vi "Save Parametric Data to csv.vi"(0 "Filepath":path=path "C:/Users/Eddie.Rickey/Desktop/Test Data", 2 "Test Information":T4={"Exp Name"="Cold Switching", "Lot"="0233A", "Wafer"="15", "Die Type"="L22", "Die X "="6", "Die Y"="8", "Exp"="1", "Die X_Y"="8"}, 3 "Parametric Calculated Values":T5={"Voltage Calculated Values"={"P1_VPD_C"=0.0, "P2_VPD_C"=0.0, "P1_VPD_Rel_C"=0.0, "P2_VPD_Rel_C"=0.0}, "Resistance Calculated Values"={"Rc_free"=0.0, "Rc_first"=0.0, "Rc_vmax"=0.0, "Rc_last"=0.0, "Rc_end"=0.0, "VPD_R"=0.0, "VPD_Rel_R"=0.0}, "Capacitance Calculated Values"={"P1_CPD_free"=0.0, "P2_CPD_free"=0.0, "P1_CPD_vmax"=0.0, "P2_CPD_vmax"=0.0, "P1_CPD_first"=0.0, "P2_CPD_first"=0.0, "P1_CPD_last"=0.0, "P2_CPD_last"=0.0, "P1_CPD_end"=0.0, "P2_CPD_end"=0.0, "P1_CPD_max"=0.0, "P2_CPD_max "=0.0, "CPD_Free"=0.0, "CPD_First"=0.0, "CPD_max"=0.0, "CPD_Last"=0.0, "CPD_End"=0.0, "CPD_vmax"=0.0}, "Cap Calc Arrays"={"CPD_sum"=[], "P2_CPD@V"=[], "P1_CPD@V"=[], "Specific Voltages"=[32.0, 36.0]}, "Resistance Array Calc"={"RC@V"=[]}, "TN4 Calc"={"P1_TN4_ACT"=0.0, "P2_TN4_ACT "=0.0, "VPD_R_2"=0.0, "DVR"=0.0}, "Corrected_Capacitance Calculated Values"={"P1_CPD_free"=0.0, "P2_CPD_free"=0.0, "P1_CPD_vmax"=0.0, "P2_CPD_vmax"=0.0, "P1_CPD_first"=0.0, "P2_CPD_first"=0.0, "P1_CPD_last"=0.0, "P2_CPD_last"=0.0, "P1_CPD_end"=0.0, "P2_CPD_end"=0.0, "P1_CPD_max"=0.0, "P2_CPD_max "=0.0, "CPD_Free"=0.0, "CPD_First"=0.0, "CPD_max"=0.0, "CPD_Last"=0.0, "CPD_End"=0.0, "CPD_vmax"=0.0}}, 4 "Date Cluster":T3, 5 "Error In":errorcluster, 6 "Cal Measurements":T1 {"Port 3 Capacitance" format="%#_6p"; "Port 2 Capacitance" format="%#_6p"; "Port 1 Capacitance" format="%#_6p"}, 8 "Additional Data":T2, 10 "Meas Type":string) -> (19 "Error Out":errorcluster)   [LabVIEW 2013]
uses:
  Controls/Parametric Calculated Values.ctl
  Controls/Voltage Calculated Values.ctl
  Controls/Resistance Individual Calculated Values.ctl
  Controls/Capacitance Individual Calculated Values.ctl
  Controls/Capacitance Array Calculated Values.ctl
  Controls/Resistance Array Calculated Values.ctl
  Controls/TN4 Calc.ctl
  Controls/Corrected_Capacitance Individual Calculated Values.ctl
  Controls/Test Information.ctl
  Controls/Date Control.ctl
  Controls/Additional Data.ctl
  Controls/ENA_Marker Measurements.ctl
  <vilib>/Utility/file.llb/Write To Spreadsheet File (string).vi
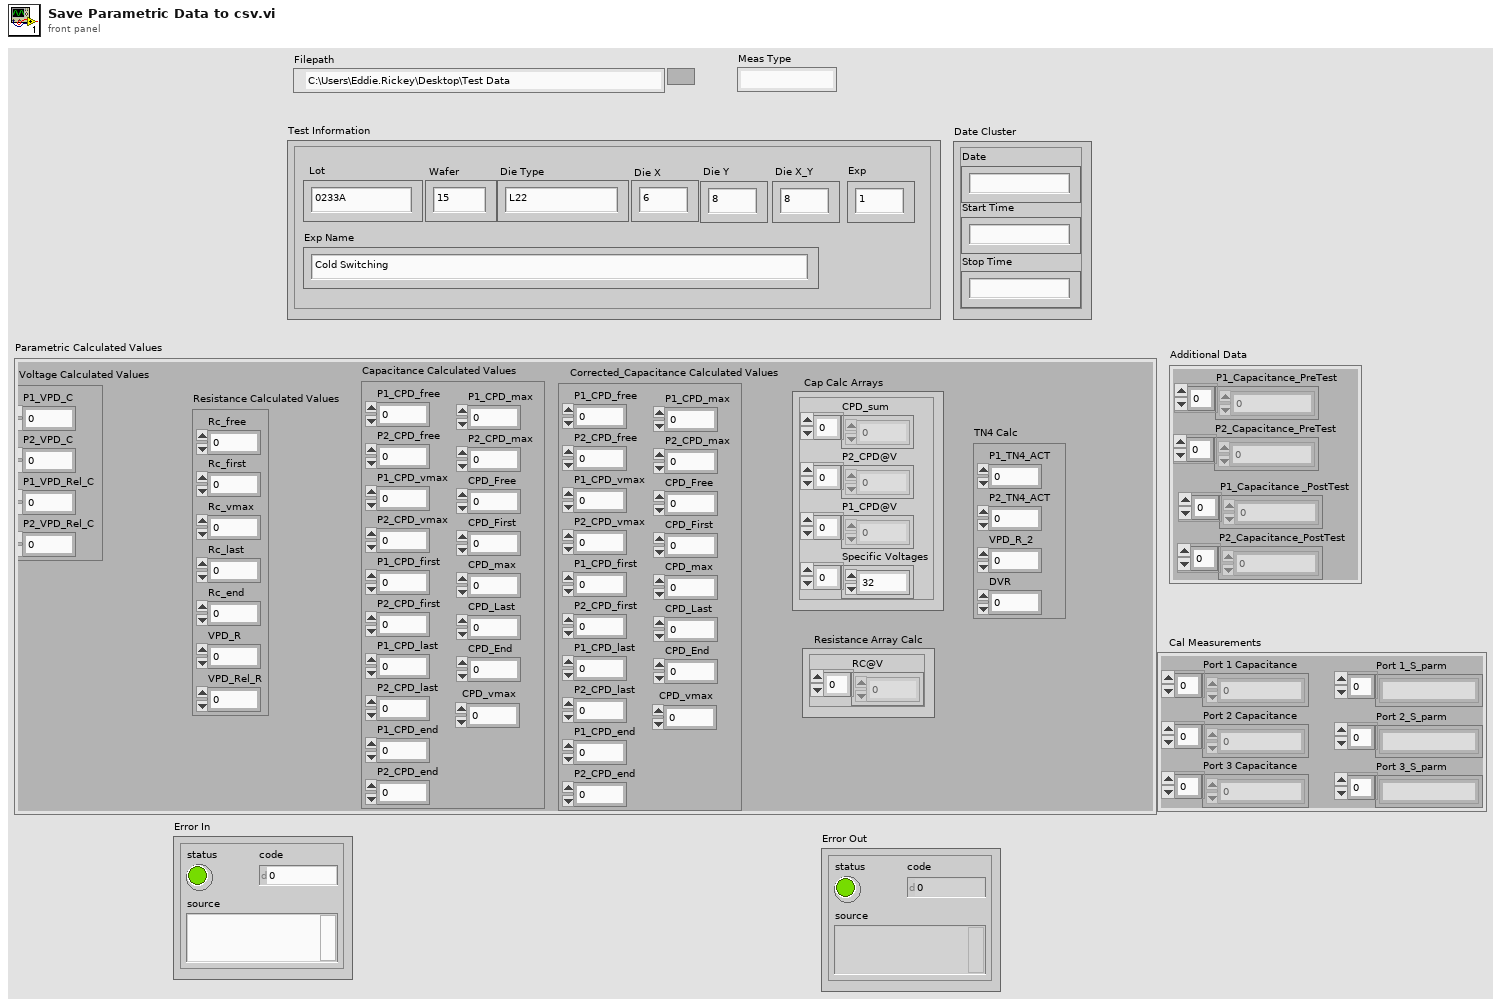
[diagram p1: front panel]
types:
  T1 = typedef "ENA_Marker Measurements.ctl" = cluster{"Port 1 Capacitance":dbl[], "Port 2 Capacitance":dbl[], "Port 3 Capacitance":dbl[], "Port 1_S_parm":string[], "Port 2_S_parm":string[], "Port 3_S_parm":string[]}
  T2 = typedef "Additional Data.ctl" = cluster{"P2_Capacitance_PostTest":dbl[], "P1_Capacitance _PostTest":dbl[], "P1_Capacitance_PreTest":dbl[], "P2_Capacitance_PreTest":dbl[]}
  T3 = typedef "Date Control.ctl" = cluster{"Date":string, "Start Time":string, "Stop Time":string}
  T4 = typedef "Test Information.ctl" = cluster{"Exp Name":string, "Lot":string, "Wafer":string, "Die Type":string, "Die X ":string, "Die Y":string, "Exp":string, "Die X_Y":string}
  T5 = typedef "Parametric Calculated Values.ctl" = cluster{"Voltage Calculated Values":T6, "Resistance Calculated Values":T7, "Capacitance Calculated Values":T8, "Cap Calc Arrays":T9, "Resistance Array Calc":T10, "TN4 Calc":T11, "Corrected_Capacitance Calculated Values":T12}
  T6 = typedef "Voltage Calculated Values.ctl" = cluster{"P1_VPD_C":dbl, "P2_VPD_C":dbl, "P1_VPD_Rel_C":dbl, "P2_VPD_Rel_C":dbl}
  T7 = typedef "Resistance Individual Calculated Values.ctl" = cluster{"Rc_free":dbl, "Rc_first":dbl, "Rc_vmax":dbl, "Rc_last":dbl, "Rc_end":dbl, "VPD_R":dbl, "VPD_Rel_R":dbl}
  T8 = typedef "Capacitance Individual Calculated Values.ctl" = cluster{"P1_CPD_free":dbl, "P2_CPD_free":dbl, "P1_CPD_vmax":dbl, "P2_CPD_vmax":dbl, "P1_CPD_first":dbl, "P2_CPD_first":dbl, "P1_CPD_last":dbl, "P2_CPD_last":dbl, "P1_CPD_end":dbl, "P2_CPD_end":dbl, "P1_CPD_max":dbl, "P2_CPD_max ":dbl, "CPD_Free":dbl, "CPD_First":dbl, "CPD_max":dbl, "CPD_Last":dbl, "CPD_End":dbl, "CPD_vmax":dbl}
  T9 = typedef "Capacitance Array Calculated Values.ctl" = cluster{"CPD_sum":dbl[], "P2_CPD@V":dbl[], "P1_CPD@V":dbl[], "Specific Voltages":dbl[]}
  T10 = typedef "Resistance Array Calculated Values.ctl" = cluster{"RC@V":dbl[]}
  T11 = typedef "TN4 Calc.ctl" = cluster{"P1_TN4_ACT":dbl, "P2_TN4_ACT ":dbl, "VPD_R_2":dbl, "DVR":dbl}
  T12 = typedef "Corrected_Capacitance Individual Calculated Values.ctl" = cluster{"P1_CPD_free":dbl, "P2_CPD_free":dbl, "P1_CPD_vmax":dbl, "P2_CPD_vmax":dbl, "P1_CPD_first":dbl, "P2_CPD_first":dbl, "P1_CPD_last":dbl, "P2_CPD_last":dbl, "P1_CPD_end":dbl, "P2_CPD_end":dbl, "P1_CPD_max":dbl, "P2_CPD_max ":dbl, "CPD_Free":dbl, "CPD_First":dbl, "CPD_max":dbl, "CPD_Last":dbl, "CPD_End":dbl, "CPD_vmax":dbl}
  T13 = enum16{"open", "replace", "create", "open or create", "replace or create", "replace or create with confirmation"}
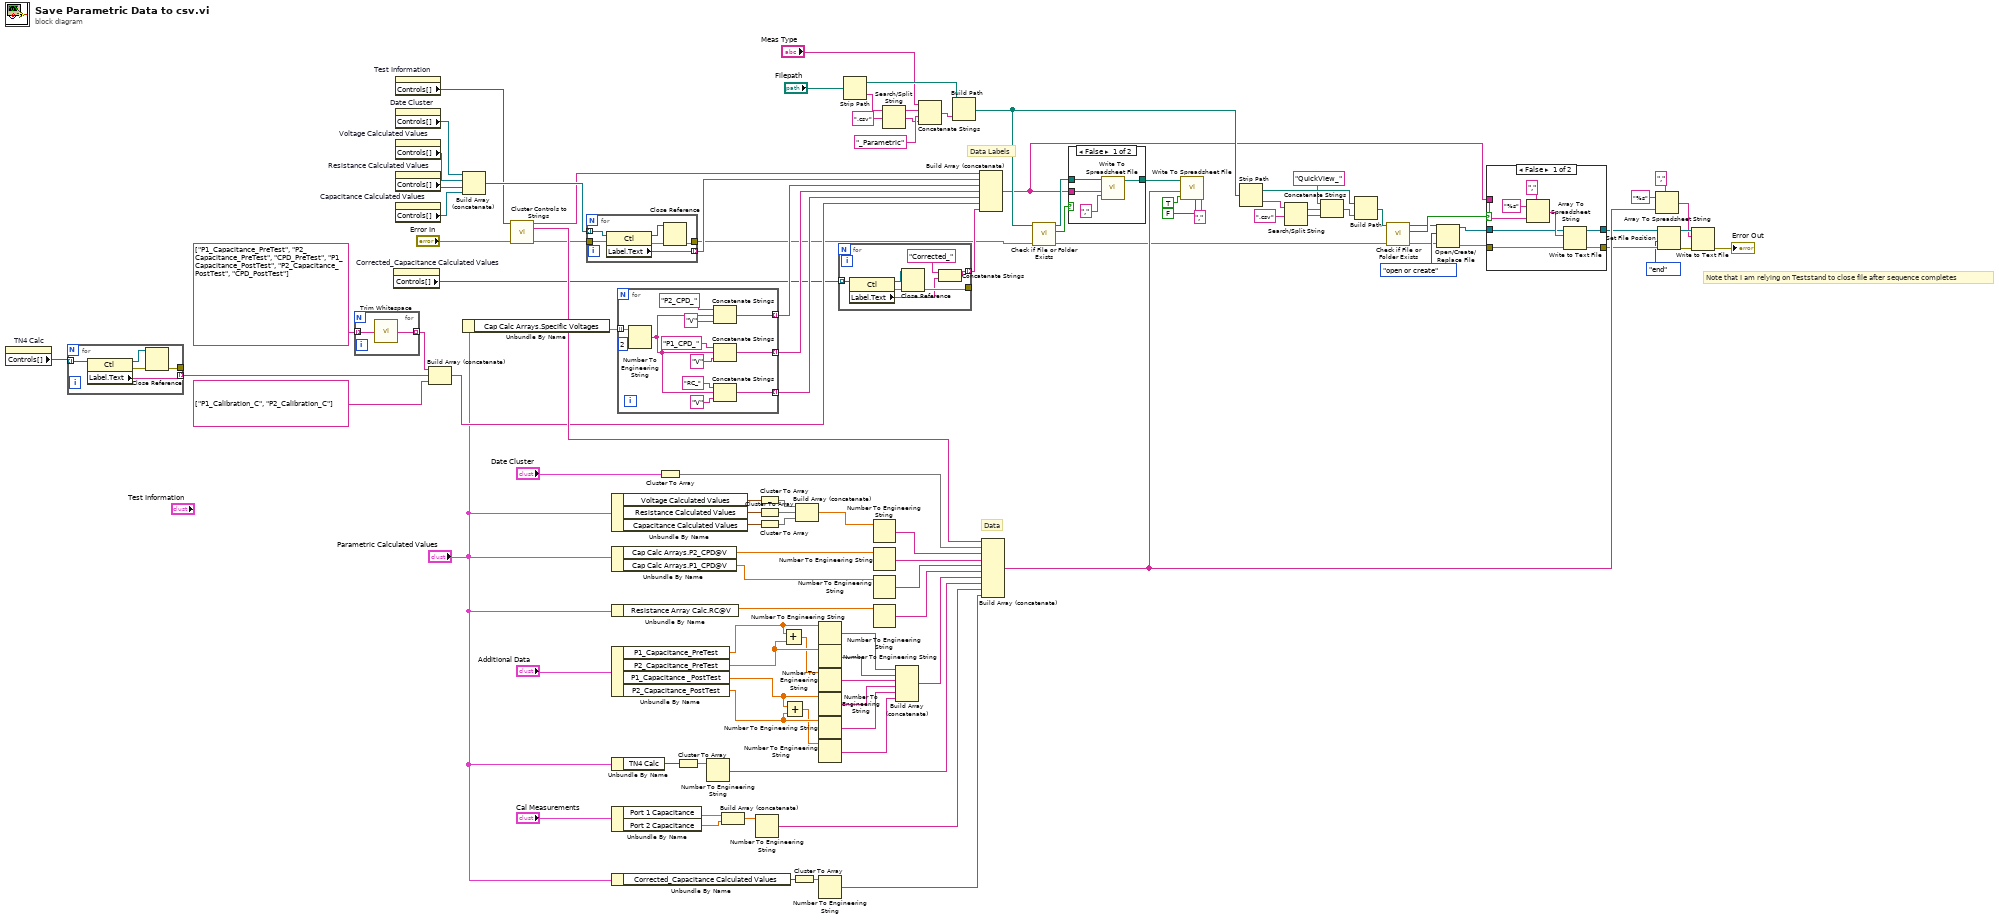
[diagram p0: block diagram]
diagram:
  # "Note that I am relying on Teststand to close file after sequence completes"
  # "Data"
  # "Data Labels"
  n1 = property on="TN4 Calc" class="Clust (strict)"() -> ("Controls[]"=w26:refnum<vi>[])  [unwired: 2 in, 2 out]
  n2 = for {
    tunnel: [w113] -> w12 mode=indexing
    tunnel: w26 -> [w112] mode=indexing
    tunnel: [w109] -> _
    n3 = property class="Ctl"(reference=w112) -> (reference out=w110:refnum<vi>, error out=w111:errorcluster, "Label.Text"=w113:string)  [unwired: 1 in]
    n4 = Close Reference(reference=w110, error in (no error)=w111) -> (error out=w109:errorcluster)
  }
  n5 = for {
    tunnel: string[] ["P1_Capacitance_PreTest", "P2_Capacitance_PreTest", "CPD_PreTest", "P1_Capacitance_PostTest", "P2_Capacitance_PostTest", "CPD_PostTest"] -> [w115] mode=indexing
    tunnel: [w114] -> w13 mode=indexing
    n6 = call <vilib>:"Trim Whitespace.vi"("string"=w115) -> ("trimmed string"=w114:string)  [unwired: 1 in]
  }
  n7 = property on="Corrected_Capacitance Calculated Values" class="Clust (strict)"() -> ("Controls[]"=w1:refnum<vi>[])  [unwired: 2 in, 2 out]
  n8 = property on="Test Information" class="Clust (strict)"() -> ("Controls[]"=w107:refnum<vi>[])  [unwired: 2 in, 2 out]
  n9 = property on="Date Cluster" class="Clust (strict)"() -> ("Controls[]"=w81:refnum<vi>[])  [unwired: 2 in, 2 out]
  n10 = property on="Voltage Calculated Values" class="Clust (strict)"() -> ("Controls[]"=w25:refnum<vi>[])  [unwired: 2 in, 2 out]
  n11 = property on="Resistance Calculated Values" class="Clust (strict)"() -> ("Controls[]"=w24:refnum<vi>[])  [unwired: 2 in, 2 out]
  n12 = property on="Capacitance Calculated Values" class="Clust (strict)"() -> ("Controls[]"=w3:refnum<vi>[])  [unwired: 2 in, 2 out]
  n13 = Build Array (concatenate)(w13, w12, string[] ["P1_Calibration_C", "P2_Calibration_C"]) -> (w14:string[])
  n14 = Build Array (concatenate)(w81, w25, w24, w3) -> (w108:refnum<vi>[])
  n15 = Unbundle By Name("Parametric Calculated Values") -> ("Cap Calc Arrays.Specific Voltages"=w89:dbl[])
  n16 = call "Cluster Controls to Strings.vi"("Controls[]"=w107, "Error In"="Error In") -> ("Control Labels"=w106:string[], "Control Values"=w80:string[], "Error Out"=w23:errorcluster)  [unwired: 11 in]
  n17 = for {
    tunnel: [w121] -> w9 mode=indexing
    tunnel: w108 -> [w120] mode=indexing
    tunnel: [w117] -> w2
    tunnel: w23 -> [w119]
    n18 = property class="Ctl"(reference=w120, error in=w119) -> (reference out=w116:refnum<vi>, error out=w118:errorcluster, "Label.Text"=w121:string)
    n19 = Close Reference(reference=w116, error in (no error)=w118) -> (error out=w117:errorcluster)
  }
  n20 = Unbundle By Name("Parametric Calculated Values") -> ("Voltage Calculated Values"=w105:T6, "Resistance Calculated Values"=w104:T7, "Capacitance Calculated Values"=w103:T8)
  n21 = Unbundle By Name("Parametric Calculated Values") -> ("Cap Calc Arrays.P2_CPD@V"=w86:dbl[], "Cap Calc Arrays.P1_CPD@V"=w85:dbl[])
  n22 = Unbundle By Name("Parametric Calculated Values") -> ("Resistance Array Calc.RC@V"=w83:dbl[])
  n23 = Unbundle By Name("Additional Data") -> ("P1_Capacitance_PreTest"=w67:dbl[], "P2_Capacitance_PreTest"=w66:dbl[], "P1_Capacitance _PostTest"=w64:dbl[], "P2_Capacitance_PostTest"=w63:dbl[])
  n24 = Unbundle By Name("Parametric Calculated Values") -> ("TN4 Calc"=w29:T11)
  n25 = Unbundle By Name("Cal Measurements") -> ("Port 1 Capacitance"=w18:dbl[], "Port 2 Capacitance"=w17:dbl[])
  n26 = Unbundle By Name("Parametric Calculated Values") -> ("Corrected_Capacitance Calculated Values"=w7:T12)
  n27 = for {
    tunnel: w89 -> [w133] mode=indexing
    tunnel: [w130] -> w90 mode=indexing
    tunnel: [w123] -> w88 mode=indexing
    tunnel: [w126] -> w87 mode=indexing
    n28 = Number To Engineering String(2:i16 2 ("precision (6)"), 4:w133) -> (0:w124:string)  [unwired: 2 in]
    n29 = Concatenate Strings("P2_CPD_" ("search string"), w124, "V" ("string")) -> (w130:string)
    n30 = Concatenate Strings("P1_CPD_" ("search string"), w124, "V" ("string")) -> (w123:string)
    n31 = Concatenate Strings("RC_" ("search string"), w124, "V" ("string")) -> (w126:string)
  }
  n32 = Cluster To Array(cluster="Date Cluster") -> (array=w78:string[])
  n33 = Cluster To Array(cluster=w29) -> (array=w28:dbl[])
  n34 = Number To Engineering String(4:w28) -> (0:w27:string[])  [unwired: 3 in]
  n35 = Build Array (concatenate)(w18, w17) -> (w16:dbl[])
  n36 = Number To Engineering String(4:w16) -> (0:w15:string[])  [unwired: 3 in]
  n37 = Cluster To Array(cluster=w105) -> (array=w102:dbl[])
  n38 = Cluster To Array(cluster=w104) -> (array=w101:dbl[])
  n39 = Cluster To Array(cluster=w103) -> (array=w10:dbl[])
  n40 = Add(x=w67, y=w66) -> (x+y=w65:dbl[])
  n41 = Add(x=w64, y=w63) -> (x+y=w62:dbl[])
  n42 = Cluster To Array(cluster=w7) -> (array=w6:dbl[])
  n43 = Build Array (concatenate)(w102, w101, w10) -> (w100:dbl[])
  n44 = Number To Engineering String(4:w67) -> (0:w61:string[])  [unwired: 3 in]
  n45 = Number To Engineering String(4:w66) -> (0:w60:string[])  [unwired: 3 in]
  n46 = Number To Engineering String(4:w65) -> (0:w59:string[])  [unwired: 3 in]
  n47 = Number To Engineering String(4:w64) -> (0:w58:string[])  [unwired: 3 in]
  n48 = Number To Engineering String(4:w63) -> (0:w57:string[])  [unwired: 3 in]
  n49 = Number To Engineering String(4:w62) -> (0:w56:string[])  [unwired: 3 in]
  n50 = Number To Engineering String(4:w6) -> (0:w5:string[])  [unwired: 3 in]
  n51 = for {
    tunnel: [w139] -> _
    tunnel: [w135] -> w4 mode=indexing
    tunnel: w1 -> [w134] mode=indexing
    n52 = property class="Ctl"(reference=w134) -> (reference out=w138:refnum<vi>, error out=w140:errorcluster, "Label.Text"=w136:string)  [unwired: 1 in]
    n53 = Close Reference(reference=w138, error in (no error)=w140) -> (error out=w139:errorcluster)
    n54 = Concatenate Strings("Corrected_" ("string"), w136) -> (w135:string)
  }
  n55 = Strip Path(path="Filepath") -> (stripped path=w92:path, name=w97:string)
  n56 = Number To Engineering String(4:w100) -> (0:w99:string[])  [unwired: 3 in]
  n57 = Number To Engineering String(4:w86) -> (0:w98:string[])  [unwired: 3 in]
  n58 = Number To Engineering String(4:w85) -> (0:w84:string[])  [unwired: 3 in]
  n59 = Number To Engineering String(4:w83) -> (0:w82:string[])  [unwired: 3 in]
  n60 = Search/Split String(string=w97, search string/char (-)=".csv" ("search string")) -> (substring before match=w95:string, match + rest of string=w93:string)  [unwired: 1 in, 1 out]
  n61 = Build Array (concatenate)(w61, w60, w59, w58, w57, w56) -> (w55:string[])
  n62 = Concatenate Strings("Meas Type", w95, "_Parametric" ("search string"), w93) -> (w91:string)
  n63 = Build Path(base path=w92, name or relative path=w91) -> (appended path=w76:path)
  n64 = Build Array (concatenate)(w106, w9, w90, w88, w87, w14, w4) -> (w70:string[])
  n65 = Build Array (concatenate)(w80, w78, w99, w98, w84, w82, w55, w27, w15, w5) -> (w69:string[])
  n66 = call <vilib>:"Check if File or Folder Exists.vi"("error in (no error)"=w2, "path"=w76) -> ("error out"=w21:errorcluster, "file or folder exists?"=w53:bool, "dup path"=w75:path)  [unwired: 7 in]
  n67 = case shown="False" w53 {
    tunnel: w75 -> [w144 w145]
    tunnel: w70 -> [w143 _]
    tunnel: [w141 w145] -> w71
    frame False {
      n68 = call-poly <vilib>:"Write To Spreadsheet File.vi"("delimiter (\\t)"="," ("delimiter (\\t)"), "1D data"=w143, "file path (dialog if empty)"=w144) -> ("new file path (Not A Path if cancelled)"=w141:path)  [unwired: 5 in]
    }
    frame True {
    }
  }
  n69 = call-poly <vilib>:"Write To Spreadsheet File.vi"("delimiter (\\t)"="," ("delimiter (\\t)"), "transpose? (no:F)"=FALSE, "append to file? (new file:F)"=TRUE, "1D data"=w69, "file path (dialog if empty)"=w71) -> ()  [unwired: 3 in, 1 out]
  n70 = Strip Path(path=w76) -> (stripped path=w46:path, name=w49:string)
  n71 = Search/Split String(string=w49, search string/char (-)=".csv" ("search string")) -> (substring before match=w44:string, match + rest of string=w47:string)  [unwired: 1 in, 1 out]
  n72 = Concatenate Strings("QuickView_" ("search string"), w44, w47) -> (w45:string)
  n73 = Build Path(base path=w46, name or relative path=w45) -> (appended path=w40:path)
  n74 = call <vilib>:"Check if File or Folder Exists.vi"("error in (no error)"=w21, "path"=w40) -> ("error out"=w39:errorcluster, "file or folder exists?"=w38:bool, "dup path"=w37:path)  [unwired: 7 in]
  n75 = Open/Create/Replace File(file path (use dialog)=w37, error in=w39, operation (0:open)=T13."open or create") -> (refnum out=w42:refnum<file>, error out=w43:errorcluster)  [unwired: 3 in, 1 out]
  n76 = case shown="False" w38 {
    tunnel: w70 -> [w151 _]
    tunnel: w42 -> [w149 w155]
    tunnel: w43 -> [w148 w154]
    tunnel: [w147 w154] -> w52
    tunnel: [w146 w155] -> w51
    frame False {
      n77 = Array To Spreadsheet String(delimiter (Tab)="," ("delimiter (\\t)"), array=w151, 3:"%s" ("format string")) -> (spreadsheet string=w150:string)
      n78 = Write to Text File(file (use dialog)=w149, text=w150, error in=w148) -> (refnum out=w146:refnum<file>, error out=w147:errorcluster)  [unwired: 1 in, 1 out]
    }
    frame True {
    }
  }
  n79 = Array To Spreadsheet String(delimiter (Tab)="," ("delimiter (\\t)"), array=w69, 3:"%s" ("format string")) -> (spreadsheet string=w31:string)
  n80 = Set File Position(refnum=w51, from (0:start)=enum16{"start", "end", "current"}."end", error in=w52) -> (refnum out=w32:refnum<file>, error out=w33:errorcluster)  [unwired: 1 in]
  n81 = Write to Text File(file (use dialog)=w32, text=w31, error in=w33) -> (error out=→"Error Out":errorcluster)  [unwired: 1 in, 2 out]
